vi "PSD_Calculation_Tom.vi"(0 "Scaled Data 1D":dbl[](array[numeric]), 1 "log/linear":enum16{"Linear", "dB", "dBm"}(ring)=enum."dB", 2 "display unit":T1(ring), 5 "Channel":i32, 7 "dt":dbl=1.0 format="%0.2f", 9 "window":T2(ring), 11 "Power Spectrum (V^2 rms)":dbl[](array[numeric]), 12 "Not 1st run?":bool, 13 "Avg completed":u32=2 min=1) -> (4 "Data from 1 channel":dbl[](array[numeric]), 6 "df":dbl format="%0.2f", 8 "Avg PSD":dbl[](array[numeric]), 10 "Spectrum out":dbl[](array[numeric]) format="%0.2f", 14 "Y Unit":string="Vrms", 15 "Power Spectrum (V^2 rms) Out":dbl[](array[numeric]))   [LabVIEW 2014]
uses:
  <vilib>/Analysis/0measdsp.llb/Scaled Time Domain Window (DBL).vi
  <vilib>/Analysis/NI_AALPro.lvlib
panel:
  in  "Scaled Data":dbl[][](array[numeric])
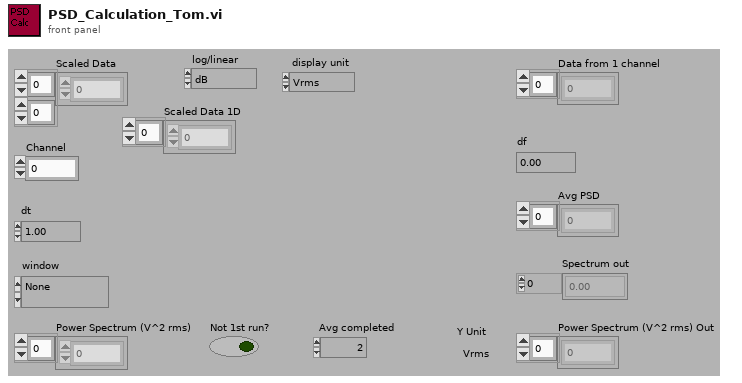
[diagram p1: front panel]
types:
  T1 = enum32{"Vrms", "Vpk", "Vrms^2", "Vpk^2", "Vrms/rtHz", "Vpk/rtHz", "Vrms^2/Hz", "Vpk^2/Hz"}
  T2 = enum16{"None ", "Hanning", "Hamming", "Blackman-Harris", "Exact Blackman", "Blackman", "Flat Top", "4 Term B-Harris ", "7 Term B-Harris", "Low Sidelobe"}
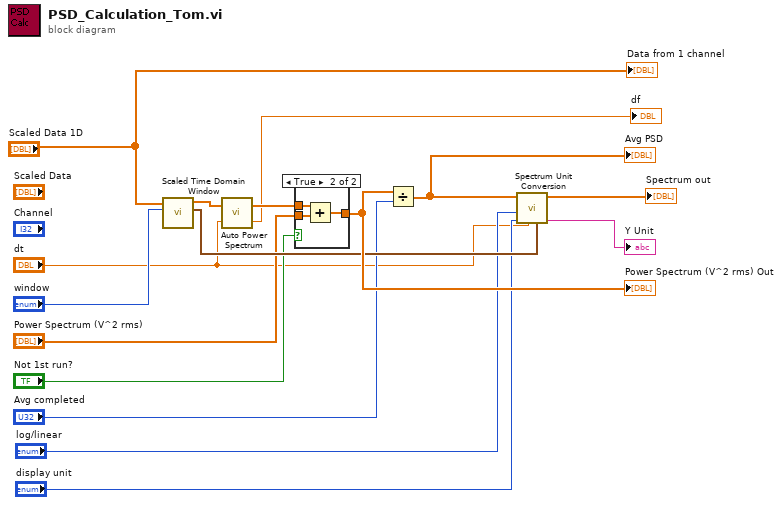
[diagram p0: block diagram]
diagram:
  n1 = call-poly <vilib>:"Scaled Time Domain Window.vi"("window"="window", "X"="Scaled Data 1D") -> ("window properties"=w12:cluster{"eq noise BW":dbl, "coherent gain":dbl}, "Windowed X"=w16:dbl[])  [unwired: 7 in, 1 out]
  n2 = call <vilib>:"Auto Power Spectrum.vi"("dt"="dt", "Signal (V)"=w16) -> ("df"=→"df":dbl, "Power Spectrum (V^2 rms)"=w15:dbl[])
  n3 = case shown="True" "Not 1st run?" {
    tunnel: w15 -> [w17 w20]
    tunnel: [w17 w18] -> w14
    tunnel: "Power Spectrum (V^2 rms)" -> [_ w19]
    frame False {
    }
    frame True {
      n4 = Add(x=w20, y=w19) -> (x+y=w18:dbl[])
    }
  }
  "Power Spectrum (V^2 rms) Out" <- w14
  n5 = Divide(x=w14, y="Avg completed") -> (x/y=w11:dbl[])
  "Avg PSD" <- w11
  n6 = call <vilib>:"Spectrum Unit Conversion.vi"("window constants"=w12, "df"="dt", "display unit"="display unit", "log/linear"="log/linear", "Spectrum in"=w11) -> ("spectrum unit"=→"Y Unit":string, "Spectrum out"=→"Spectrum out":dbl[])  [unwired: 5 in]
  "Data from 1 channel" <- "Scaled Data 1D"
